vi "Begin.vi"() -> (0 "CameraDevRef 2":T1, 1 "CameraDevRef":T1)   [LabVIEW 2011]
doc: "Called before other user functions, this VI is expected to open initial I/O refnums, load in file data, and do all program initialization. Notice that the <B>error out</B> terminal is simply used for data flow. Wiring it to other structures or subVIs ensures that this VI runs first."
uses:
  <vilib>/Rock Robotics/WPI/Camera/WPI_CameraDevRef.ctl
  <vilib>/Rock Robotics/SystemInterfaces/DIO/FPGA_DIOPWMChannel.ctl
  <vilib>/Rock Robotics/WPI/Joystick/WPI_JoystickDeviceEnum.ctl
  <vilib>/Rock Robotics/SystemInterfaces/AI/FPGA_AIChannel.ctl
  <vilib>/Rock Robotics/SystemInterfaces/DIO/FPGA_DIORelayChannel.ctl
  <vilib>/Rock Robotics/SystemInterfaces/DIO/FPGA_DIOChannel.ctl
  <vilib>/Rock Robotics/SystemInterfaces/AI/FPGA_AIGyroChannel.ctl
  <vilib>/Rock Robotics/WPI/Relay/WPI_RelayDirection.ctl
  <vilib>/Rock Robotics/WPI/Encoder/WPI_EncoderType.ctl
  <vilib>/Rock Robotics/WPI/MotorControl/WPI_MotorControlOpen Victor.vi
  <vilib>/Rock Robotics/WPI/MotorControl/WPI_MotorControlOpen Jaguar.vi
  Robot Global Data.vi
  <vilib>/Utility/file.llb/Read From Spreadsheet File (DBL).vi
  <vilib>/Rock Robotics/WPI/Counter/WPI_CounterDigitalInputToDigitalSource.vi
  <vilib>/Rock Robotics/SystemInterfaces/Typedef/FPGA_TypedefDigitalModule.ctl
  <vilib>/Rock Robotics/SystemInterfaces/Typedef/FPGA_TypedefAnalogModule.ctl
panel:
  out "Path and file":string
  in  "Balls In Robot At Start":dbl=2.0
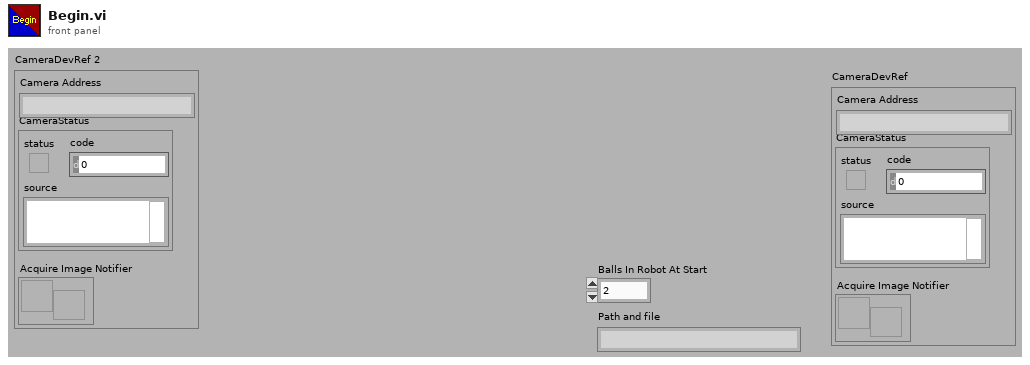
[diagram p1: front panel]
types:
  T1 = typedef "WPI_CameraDevRef.ctl" = cluster{"Camera Address":string, "CameraStatus":errorcluster, "Acquire Image Notifier":refnum<notifier>}
  T2 = typedef "WPI_EncoderType.ctl" = enum16{"1x", "2x", "4x"}
  T3 = typedef "FPGA_DIOChannel.ctl" = enum8{"DIO 1", "DIO 2", "DIO 3", "DIO 4", "DIO 5", "DIO 6", "DIO 7", "DIO 8", "DIO 9", "DIO 10", "DIO 11", "DIO 12", "DIO 13", "DIO 14", "Invalid"}
  T4 = typedef "FPGA_DIORelayChannel.ctl" = enum8{"Relay 1", "Relay 2", "Relay 3", "Relay 4", "Relay 5", "Relay 6", "Relay 7", "Relay 8", "Invalid"}
  T5 = typedef "WPI_RelayDirection.ctl" = enum16{"Both directions", "Forward only", "Reverse only"}
  T6 = typedef "FPGA_AIGyroChannel.ctl" = enum8{"AI 1", "AI 2", "Invalid"}
  T7 = typedef "FPGA_DIOPWMChannel.ctl" = enum8{"PWM 1", "PWM 2", "PWM 3", "PWM 4", "PWM 5", "PWM 6", "PWM 7", "PWM 8", "PWM 9", "PWM 10", "Invalid"}
  T8 = typedef "FPGA_AIChannel.ctl" = enum8{"AI 1", "AI 2", "AI 3", "AI 4", "AI 5", "AI 6", "AI 7", "AI 8", "Invalid"}
  T9 = typedef "WPI_JoystickDeviceEnum.ctl" = enum16{"USB 1", "USB 2", "USB 3", "USB 4", "Kinect 1", "Kinect 2"}
  T10 = typedef "WPI_CameraImageSize.ctl" = enum16{"640x480", "320x240", "160x120"}
  T11 = cluster{"fps":i32, "compression":i32, "Image Size":T10}
  T12 = typedef "WPI_MotorControlDeviceRef.ctl" = cluster{"DeviceStatus":errorcluster, "Type":enum16{"PWM", "CAN"}, "PWM":cluster{"Digital Module":T13, "PWM Channel":T7, "DeadBand":T14}, "CAN":cluster{"Device Number":u8, "Control Mode":T15, "Semaphore":T16, "Max Vout":dbl}, "Invert":bool, "TransformRef":T17, "InvTransformRef":T17}
  T13 = typedef "FPGA_TypedefDigitalModule.ctl" = enum16{"Digital Module 1", "Digital Module 2"}
  T14 = typedef "WPI_PWMDeadband.ctl" = cluster{"Name":string, "maxPositivePwm":i32, "minPositivePwm":i32, "centerPwm":i32, "maxNegativePwm":i32, "minNegativePwm":i32, "angularRange":u16}
  T15 = typedef "WPI_CANJaguar_ControlMode.ctl" = enum8{"Percent VBus", "Current", "Speed", "Position", "Voltage"}
  T16 = typedef "Semaphore RefNum" = refnum<k1>
  T17 = typedef "WPI_PWMTransform_ConPane.ctl" = refnum<vi>
  T18 = typedef "WPI_ServoDeviceRef.ctl" = cluster{"DeviceStatus":errorcluster, "Digital Module":T13, "PWM Channel":T7, "DeadBand":T14}
  T19 = typedef "WPI_AnalogChannelDevRef.ctl" = cluster{"DevStatus":errorcluster, "Analog Module":T20, "Analog Channel":T8}
  T20 = typedef "FPGA_TypedefAnalogModule.ctl" = enum16{"Analog Module 1", "Analog Module 2"}
  T21 = typedef "WPI_CameraWhite Balance Values.ctl" = enum16{"Auto", "Fixed indoor", "Fixed outdoor 1", "Fixed outdoor 2", "Fixed fluorescent 1", "Fixed fluorescent 2", "Hold current"}
  T22 = typedef "WPI_JoystickDevRef.ctl" = cluster{"Device":T9}
  T23 = typedef "WPI_RelayDevRef.ctl" = cluster{"DevStatus":errorcluster, "Relay Channel":T4, "Digital Module":T13, "Relay Direction":T5}
  T24 = typedef "WPI_CameraExposure Values.ctl" = enum16{"Auto", "Flicker-free 50 Hz", "Flicker-free 60 Hz", "Hold current"}
  T25 = typedef "WPI_DigitalInputDevRef.ctl" = cluster{"DevStatus":errorcluster, "DIO Channel":T3, "Digital Module":T13}
  T26 = typedef "FPGA_CounterEncoderSourceConvertionLVSourceType.ctl" = cluster{"DevStatus":errorcluster, "AnalogTriggerMode?":bool, "DigitalMode":cluster{"Digital Module":T13, "DIO Channel":T27}, "AnalogTriggerMode":cluster{"AnalogTriggerIndex":T28, "OutputType":T29}}
  T27 = typedef "FPGA_DIODigitalSourceChannel.ctl" = enum8{"DIO 1", "DIO 2", "DIO 3", "DIO 4", "DIO 5", "DIO 6", "DIO 7", "DIO 8", "DIO 9", "DIO 10", "DIO 11", "DIO 12", "DIO 13", "DIO 14", "Disabled"}
  T28 = typedef "FPGA_AnalogTriggerIndex.ctl" = enum8{"Trig 0", "Trig 1", "Trig 2", "Trig 3", "Trig 4", "Trig 5", "Trig 6", "Trig 7", "Invalid"}
  T29 = typedef "FPGA_AnalogTriggerOutType.ctl" = enum16{"InWindow", "TriggerState", "Rising", "Falling"}
  T30 = typedef "WPI_EncoderDevRef.ctl" = cluster{"DevStatus":errorcluster, "EncoderIndex":T31, "CounterIndex":T32, "DistancePerCount":dbl, "Decoding Type":T2}
  T31 = typedef "FPGA_EncoderIdx.ctl" = enum8{"Enc 0", "Enc 1", "Enc 2", "Enc 3", "Invalid"}
  T32 = typedef "FPGA_CounterCtrSystemIndex.ctl" = enum8{"Ctr 0", "Ctr 1", "Ctr 2", "Ctr 3", "Ctr 4", "Ctr 5", "Ctr 6", "Ctr 7", "Invalid"}
  T33 = typedef "WPI_GyroDevRef.ctl" = cluster{"DevStatus":errorcluster, "Analog Module":T20, "Analog Channel":T8, "Offset":dbl, "Gain (VoltsPerDegree/Second)":dbl}
  T34 = typedef "WPI_UltrasonicDeviceRef.ctl" = cluster{"DevStatus":errorcluster, "Ping Digital Module":T13, "Echo Digital Module":T13, "Ping Channel":T3, "Echo Channel":T3, "CntIndex":T32}
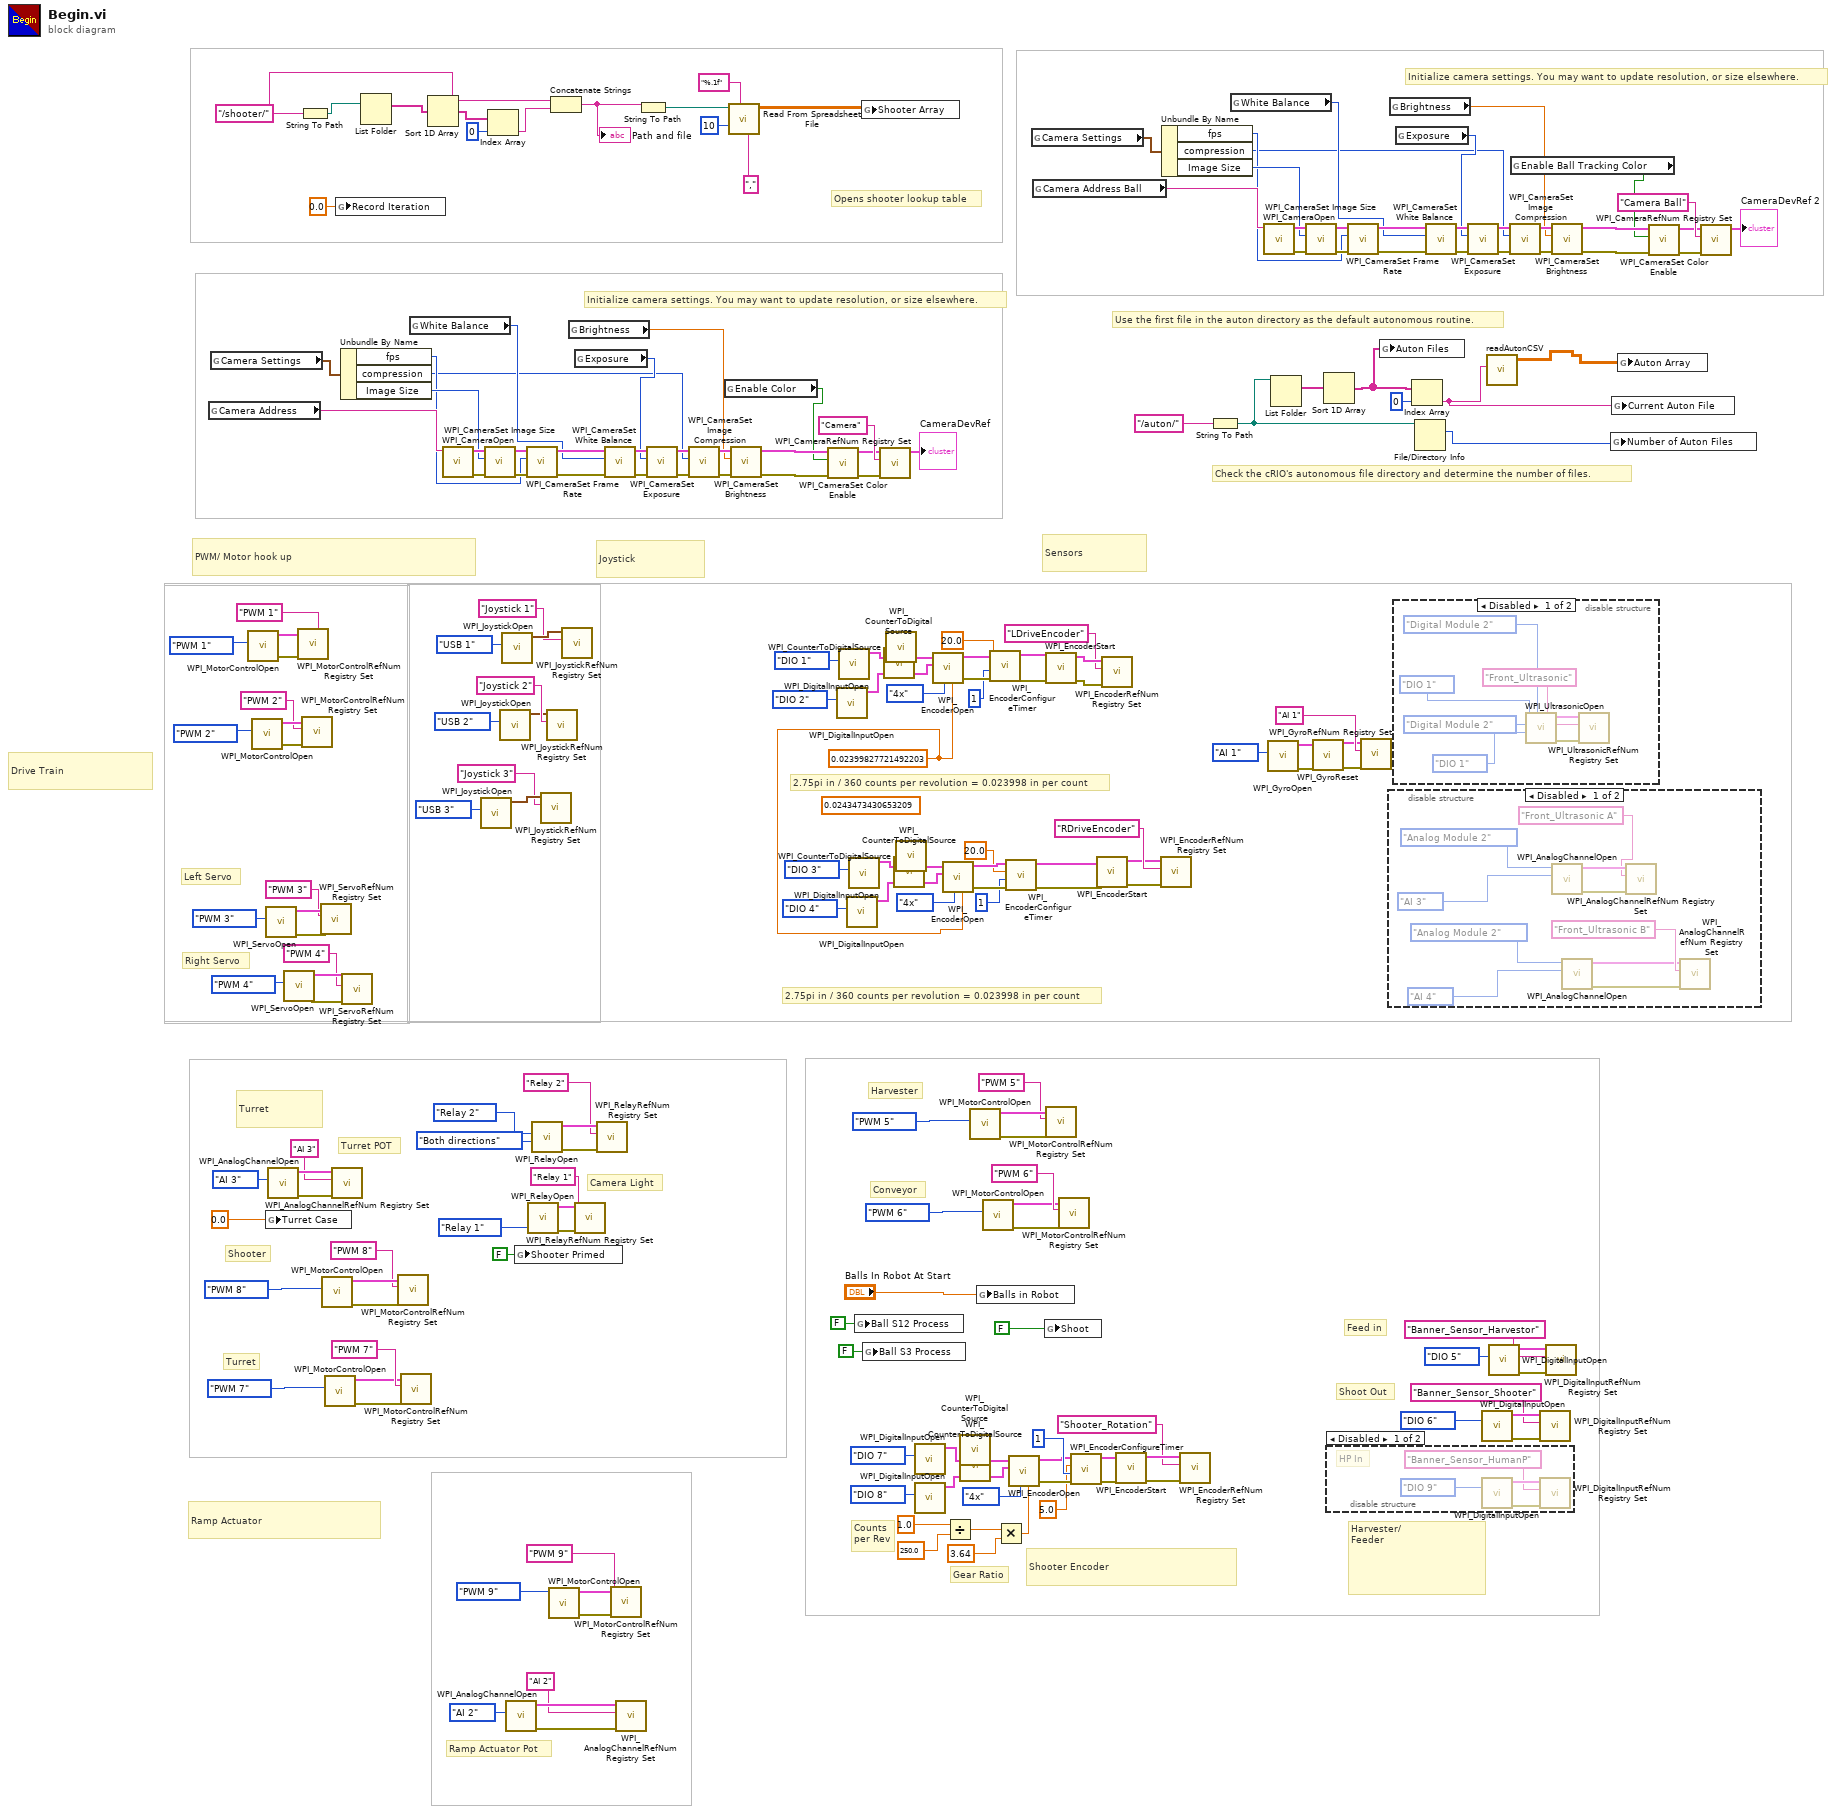
[diagram p0: block diagram]
diagram:
  (unwired) 0.0243473430653209 ("DistancePerCount")
  w49 = 0.02399827721492203 ("DistancePerCount")
  w99 = "/shooter/" ("string")
  # "Shooter Encoder"
  # "Counts\nper Rev"
  # "Gear Ratio"
  # "Initialize camera settings. You may want to update resolution, or size elsewhere."
  # "Check the cRIO's autonomous file directory and determine the number of files."
  # "Use the first file in the auton directory as the default autonomous routine."
  # "2.75pi in / 360 counts per revolution = 0.023998 in per count"
  # "2.75pi in / 360 counts per revolution = 0.023998 in per count"
  # "Opens shooter lookup table"
  # "Shoot Out"
  # "Feed in"
  # "Harvester"
  # "Conveyor"
  # "Shooter"
  # "Initialize camera settings. You may want to update resolution, or size elsewhere."
  # "Camera Light"
  # "Ramp Actuator Pot"
  # "Turret POT"
  # "Turret"
  # "Right Servo"
  # "Left Servo"
  # "Harvester/\nFeeder"
  # "Turret"
  # "Ramp Actuator"
  # "Drive Train"
  # "Sensors"
  # "Joystick"
  # "PWM/ Motor hook up"
  n1 = global read "Robot Global Data.vi" "Camera Address"() -> (w152:string)
  n2 = global read "Robot Global Data.vi" "Camera Settings"() -> (w151:T11)
  n3 = call-poly <vilib>:"WPI_MotorControlOpen.vi"("PWM Channel"=FPGA_DIOPWMChannel."PWM 1") -> ("error out"=w192:errorcluster, "MotorControlDeviceRef"=w194:T12)  [unwired: 9 in]
  n4 = call-poly <vilib>:"WPI_MotorControlOpen.vi"("PWM Channel"=FPGA_DIOPWMChannel."PWM 2") -> ("error out"=w190:errorcluster, "MotorControlDeviceRef"=w188:T12)  [unwired: 9 in]
  n5 = call <vilib>:"WPI_ServoOpen.vi"("PWM Channel"=FPGA_DIOPWMChannel."PWM 3") -> ("error out"=w205:errorcluster, "ServoDeviceRef"=w210:T18)  [unwired: 9 in]
  n6 = global write "Robot Global Data.vi" "Turret Case"(0.0 ("Return To Home Case")) -> ()
  n7 = call <vilib>:"WPI_AnalogChannelOpen.vi"("Analog Channel"=FPGA_AIChannel."AI 3") -> ("error out"=w181:errorcluster, "AIDeviceRef"=w182:T19)  [unwired: 9 in]
  n8 = call <vilib>:"WPI_ServoOpen.vi"("PWM Channel"=FPGA_DIOPWMChannel."PWM 4") -> ("error out"=w204:errorcluster, "ServoDeviceRef"=w208:T18)  [unwired: 9 in]
  n9 = call <vilib>:"WPI_MotorControlRefNum Registry Set.vi"("error in (no error)"=w192, "refnum name"="PWM 1", "MotorControlDevRef"=w194) -> ()  [unwired: 7 in, 2 out]
  n10 = String To Path(string=w99) -> (path=w108:path)
  n11 = call <vilib>:"WPI_MotorControlRefNum Registry Set.vi"("error in (no error)"=w190, "refnum name"="PWM 2", "MotorControlDevRef"=w188) -> ()  [unwired: 7 in, 2 out]
  n12 = call <vilib>:"WPI_ServoRefNum Registry Set.vi"("error in (no error)"=w205, "refnum name"="PWM 3", "ServoDeviceRef"=w210) -> ()  [unwired: 7 in, 2 out]
  n13 = call-poly <vilib>:"WPI_MotorControlOpen.vi"("PWM Channel"=FPGA_DIOPWMChannel."PWM 8") -> ("error out"=w135:errorcluster, "MotorControlDeviceRef"=w137:T12)  [unwired: 9 in]
  n14 = call-poly <vilib>:"WPI_MotorControlOpen.vi"("PWM Channel"=FPGA_DIOPWMChannel."PWM 7") -> ("error out"=w186:errorcluster, "MotorControlDeviceRef"=w184:T12)  [unwired: 9 in]
  n15 = call <vilib>:"WPI_AnalogChannelRefNum Registry Set.vi"("error in (no error)"=w181, "refnum name"="AI 3", "AIDeviceRef"=w182) -> ()  [unwired: 7 in, 2 out]
  n16 = global write "Robot Global Data.vi" "Record Iteration"(0.0 ("Record Iteration")) -> ()
  n17 = Unbundle By Name(w151) -> ("fps"=w149:i32, "compression"=w146:i32, "Image Size"=w150:T10)
  n18 = call <vilib>:"WPI_ServoRefNum Registry Set.vi"("error in (no error)"=w204, "refnum name"="PWM 4", "ServoDeviceRef"=w208) -> ()  [unwired: 7 in, 2 out]
  n19 = List Folder(path=w108) -> (filenames=w107:string[])  [unwired: 1 in, 5 out]
  n20 = call <vilib>:"WPI_MotorControlRefNum Registry Set.vi"("error in (no error)"=w135, "refnum name"="PWM 8", "MotorControlDevRef"=w137) -> ()  [unwired: 7 in, 2 out]
  n21 = call <vilib>:"WPI_MotorControlRefNum Registry Set.vi"("error in (no error)"=w186, "refnum name"="PWM 7", "MotorControlDevRef"=w184) -> ()  [unwired: 7 in, 2 out]
  n22 = global read "Robot Global Data.vi" "White Balance"() -> (w148:T21)
  n23 = Sort 1D Array(array=w107) -> (sorted array=w106:string[])
  n24 = call <vilib>:"WPI_CameraOpen.vi"("Camera Address"=w152) -> ("error out"=w158:errorcluster, "CameraDevRef"=w159:T1)  [unwired: 1 in, 8 out]
  n25 = call <vilib>:"WPI_JoystickOpen.vi"("JoystickDevice"=WPI_JoystickDeviceEnum."USB 3") -> ("JoystickDevRef"=w197:T22)  [unwired: 10 in]
  n26 = call <vilib>:"WPI_CameraSet Image Size.vi"("error in (no error)"=w158, "Image Size"=w150, "CameraDevRef"=w159) -> ("error out"=w157:errorcluster, "CameraDevRef Out"=w160:T1)  [unwired: 7 out]
  n27 = Index Array(array=w106, index=0) -> (element=w98:string)
  n28 = call <vilib>:"WPI_JoystickOpen.vi"("JoystickDevice"=WPI_JoystickDeviceEnum."USB 2") -> ("JoystickDevRef"=w200:T22)  [unwired: 10 in]
  n29 = call <vilib>:"WPI_JoystickOpen.vi"("JoystickDevice"=WPI_JoystickDeviceEnum."USB 1") -> ("JoystickDevRef"=w203:T22)  [unwired: 10 in]
  n30 = call <vilib>:"WPI_AnalogChannelOpen.vi"("Analog Channel"=FPGA_AIChannel."AI 2") -> ("error out"=w176:errorcluster, "AIDeviceRef"=w177:T19)  [unwired: 9 in]
  n31 = global write "Robot Global Data.vi" "Shooter Primed"(FALSE ("Ball S3 Process")) -> ()
  n32 = call <vilib>:"WPI_CameraSet Frame Rate.vi"("error in (no error)"=w157, "Frame Rate (fps)"=w149, "CameraDevRef"=w160) -> ("error out"=w156:errorcluster, "CameraDevRef Out"=w162:T1)  [unwired: 7 out]
  n33 = call <vilib>:"WPI_RelayOpen.vi"("Relay Channel"=FPGA_DIORelayChannel."Relay 1") -> ("error out"=w169:errorcluster, "RelayDevRef"=w168:T23)  [unwired: 9 in]
  n34 = call <vilib>:"WPI_RelayOpen.vi"("Relay Direction"=WPI_RelayDirection."Both directions", "Relay Channel"=FPGA_DIORelayChannel."Relay 2") -> ("error out"=w93:errorcluster, "RelayDevRef"=w94:T23)  [unwired: 8 in]
  n35 = call <vilib>:"WPI_JoystickRefNum Registry Set.vi"("refnum name"="Joystick 3", "JoystickDevRef"=w197) -> ()  [unwired: 8 in, 2 out]
  n36 = call <vilib>:"WPI_JoystickRefNum Registry Set.vi"("refnum name"="Joystick 2", "JoystickDevRef"=w200) -> ()  [unwired: 8 in, 2 out]
  n37 = call-poly <vilib>:"WPI_MotorControlOpen.vi"("PWM Channel"=FPGA_DIOPWMChannel."PWM 9") -> ("error out"=w172:errorcluster, "MotorControlDeviceRef"=w173:T12)  [unwired: 9 in]
  n38 = Concatenate Strings(w99, w98) -> (w101:string)
  "Path and file" <- w101
  n39 = call <vilib>:"WPI_JoystickRefNum Registry Set.vi"("refnum name"="Joystick 1", "JoystickDevRef"=w203) -> ()  [unwired: 8 in, 2 out]
  n40 = global read "Robot Global Data.vi" "Brightness"() -> (w145:dbl)
  n41 = global read "Robot Global Data.vi" "Exposure"() -> (w147:T24)
  n42 = call <vilib>:"WPI_RelayRefNum Registry Set.vi"("error in (no error)"=w169, "refnum name"="Relay 1", "RelayDevRef"=w168) -> ()  [unwired: 7 in, 2 out]
  n43 = call <vilib>:"WPI_RelayRefNum Registry Set.vi"("error in (no error)"=w93, "refnum name"="Relay 2", "RelayDevRef"=w94) -> ()  [unwired: 7 in, 2 out]
  n44 = call <vilib>:"WPI_CameraSet White Balance.vi"("error in (no error)"=w156, "White Balance"=w148, "CameraDevRef"=w162) -> ("error out"=w155:errorcluster, "CameraDevRef Out"=w161:T1)  [unwired: 7 out]
  n45 = call <vilib>:"WPI_MotorControlRefNum Registry Set.vi"("error in (no error)"=w172, "refnum name"="PWM 9", "MotorControlDevRef"=w173) -> ()  [unwired: 7 in, 2 out]
  n46 = call <vilib>:"WPI_AnalogChannelRefNum Registry Set.vi"("error in (no error)"=w176, "refnum name"="AI 2", "AIDeviceRef"=w177) -> ()  [unwired: 7 in, 2 out]
  n47 = String To Path(string=w101) -> (path=w100:path)
  n48 = call <vilib>:"WPI_CameraSet Exposure.vi"("error in (no error)"=w155, "Exposure"=w147, "CameraDevRef"=w161) -> ("error out"=w154:errorcluster, "CameraDevRef Out"=w164:T1)  [unwired: 7 out]
  n49 = call <vilib>:"WPI_CameraSet Image Compression.vi"("error in (no error)"=w154, "Compression"=w146, "CameraDevRef"=w164) -> ("error out"=w153:errorcluster, "CameraDevRef Out"=w163:T1)  [unwired: 7 out]
  n50 = global read "Robot Global Data.vi" "Enable Color"() -> (w140:bool)
  n51 = call-poly <vilib>:"Read From Spreadsheet File.vi"("delimiter (\\t)"="," ("delimiter (\\t)"), "format (%.3f)"="%.1f", "number of rows (all:-1)"=10, "file path (dialog if empty)"=w100) -> ("all rows"=w97:dbl[][])  [unwired: 1 in, 6 out]
  n52 = call <vilib>:"WPI_CameraSet Brightness.vi"("error in (no error)"=w153, "Brightness"=w145, "CameraDevRef"=w163) -> ("error out"=w143:errorcluster, "CameraDevRef Out"=w144:T1)  [unwired: 7 out]
  n53 = call <vilib>:"WPI_CameraSet Color Enable.vi"("error in (no error)"=w143, "Color Enabled"=w140, "CameraDevRef"=w144) -> ("error out"=w141:errorcluster, "CameraDevRef Out"=w142:T1)  [unwired: 7 in]
  n54 = call <vilib>:"WPI_DigitalInputOpen.vi"("DIO Channel"=FPGA_DIOChannel."DIO 2") -> ("DigitalInputDevRef"=w85:T25)  [unwired: 9 in, 1 out]
  n55 = call <vilib>:"WPI_DigitalInputOpen.vi"("DIO Channel"=FPGA_DIOChannel."DIO 1") -> ("DigitalInputDevRef"=w82:T25)  [unwired: 9 in, 1 out]
  n56 = call <vilib>:"WPI_DigitalInputOpen.vi"("DIO Channel"=FPGA_DIOChannel."DIO 4") -> ("DigitalInputDevRef"=w76:T25)  [unwired: 9 in, 1 out]
  n57 = call <vilib>:"WPI_DigitalInputOpen.vi"("DIO Channel"=FPGA_DIOChannel."DIO 3") -> ("DigitalInputDevRef"=w79:T25)  [unwired: 9 in, 1 out]
  n58 = global write "Robot Global Data.vi" "Ball S12 Process"(FALSE ("Ball S12 Process")) -> ()
  n59 = global write "Robot Global Data.vi" "Shooter Array"(w97) -> ()
  n60 = global write "Robot Global Data.vi" "Ball S3 Process"(FALSE ("Ball S3 Process")) -> ()
  n61 = call <vilib>:"WPI_CameraRefNum Registry Set.vi"("error in (no error)"=w141, "refnum name"="Camera", "CameraDevRef"=w142) -> ("CameraDevRef"=→"CameraDevRef":T1)  [unwired: 8 out]
  n62 = call-poly <vilib>:"WPI_CounterToDigitalSource.vi"("DigitalInputDevRef"=w85) -> ("Digital Source"=w86:T26)  [unwired: 6 in]
  n63 = call-poly <vilib>:"WPI_CounterToDigitalSource.vi"("DigitalInputDevRef"=w82) -> ("Digital Source"=w81:T26)  [unwired: 6 in]
  n64 = call-poly <vilib>:"WPI_CounterToDigitalSource.vi"("DigitalInputDevRef"=w76) -> ("Digital Source"=w75:T26)  [unwired: 6 in]
  n65 = call-poly <vilib>:"WPI_CounterToDigitalSource.vi"("DigitalInputDevRef"=w79) -> ("Digital Source"=w80:T26)  [unwired: 6 in]
  n66 = call <vilib>:"WPI_DigitalInputOpen.vi"("DIO Channel"=FPGA_DIOChannel."DIO 7") -> ("DigitalInputDevRef"=w33:T25)  [unwired: 9 in, 1 out]
  n67 = call <vilib>:"WPI_DigitalInputOpen.vi"("DIO Channel"=FPGA_DIOChannel."DIO 8") -> ("DigitalInputDevRef"=w36:T25)  [unwired: 9 in, 1 out]
  n68 = call <vilib>:"WPI_EncoderOpen.vi"("DistancePerCount"=w49, "Decoding Type"=WPI_EncoderType."4x", "BSource"=w86, "ASource"=w81) -> ("error out"=w53:errorcluster, "EncoderDevRef"=w56:T30)  [unwired: 6 in]
  n69 = call <vilib>:"WPI_EncoderOpen.vi"("DistancePerCount"=w49, "Decoding Type"=WPI_EncoderType."4x", "BSource"=w75, "ASource"=w80) -> ("error out"=w72:errorcluster, "EncoderDevRef"=w71:T30)  [unwired: 6 in]
  n70 = Divide(x=1.0, y=250.0) -> (x/y=w30:dbl)
  n71 = call-poly <vilib>:"WPI_CounterToDigitalSource.vi"("DigitalInputDevRef"=w33) -> ("Digital Source"=w32:T26)  [unwired: 6 in]
  n72 = call-poly <vilib>:"WPI_CounterToDigitalSource.vi"("DigitalInputDevRef"=w36) -> ("Digital Source"=w37:T26)  [unwired: 6 in]
  n73 = call-poly <vilib>:"WPI_MotorControlOpen.vi"("PWM Channel"=FPGA_DIOPWMChannel."PWM 5") -> ("error out"=w131:errorcluster, "MotorControlDeviceRef"=w133:T12)  [unwired: 9 in]
  n74 = global write "Robot Global Data.vi" "Balls in Robot"("Balls In Robot At Start") -> ()
  n75 = call-poly <vilib>:"WPI_MotorControlOpen.vi"("PWM Channel"=FPGA_DIOPWMChannel."PWM 6") -> ("error out"=w130:errorcluster, "MotorControlDeviceRef"=w128:T12)  [unwired: 9 in]
  n76 = call <vilib>:"WPI_EncoderConfigureTimer.vi"("error in (no error)"=w53, "Number Samples to Average"=u8 1, "Minimum Rate"=20.0, "EncoderDevRef"=w56) -> ("error out"=w54:errorcluster, "EncoderDevRef"=w55:T30)  [unwired: 6 in]
  n77 = Multiply(x=w30, y=3.64) -> (x*y=w28:dbl)
  n78 = call <vilib>:"WPI_EncoderConfigureTimer.vi"("error in (no error)"=w72, "Number Samples to Average"=u8 1, "Minimum Rate"=20.0, "EncoderDevRef"=w71) -> ("error out"=w68:errorcluster, "EncoderDevRef"=w69:T30)  [unwired: 6 in]
  n79 = call <vilib>:"WPI_EncoderOpen.vi"("DistancePerCount"=w28, "Decoding Type"=WPI_EncoderType."4x", "BSource"=w37, "ASource"=w32) -> ("error out"=w40:errorcluster, "EncoderDevRef"=w41:T30)  [unwired: 6 in]
  n80 = global read "Robot Global Data.vi" "Camera Settings"() -> (w13:T11)
  n81 = global read "Robot Global Data.vi" "Camera Address Ball"() -> (w14:string)
  n82 = global write "Robot Global Data.vi" "Shoot"(FALSE ("Ball S12 Process")) -> ()
  n83 = call <vilib>:"WPI_EncoderStart.vi"("error in (no error)"=w54, "EncoderDevRef"=w55) -> ("error out"=w89:errorcluster, "EncoderDevRef"=w88:T30)  [unwired: 8 in]
  n84 = call <vilib>:"WPI_MotorControlRefNum Registry Set.vi"("error in (no error)"=w131, "refnum name"="PWM 5", "MotorControlDevRef"=w133) -> ()  [unwired: 7 in, 2 out]
  n85 = call <vilib>:"WPI_MotorControlRefNum Registry Set.vi"("error in (no error)"=w130, "refnum name"="PWM 6", "MotorControlDevRef"=w128) -> ()  [unwired: 7 in, 2 out]
  n86 = call <vilib>:"WPI_EncoderConfigureTimer.vi"("error in (no error)"=w40, "Number Samples to Average"=u8 1, "Minimum Rate"=5.0, "EncoderDevRef"=w41) -> ("error out"=w44:errorcluster, "EncoderDevRef"=w43:T30)  [unwired: 6 in]
  n87 = call <vilib>:"WPI_EncoderStart.vi"("error in (no error)"=w68, "EncoderDevRef"=w69) -> ("error out"=w66:errorcluster, "EncoderDevRef"=w67:T30)  [unwired: 8 in]
  n88 = call <vilib>:"WPI_EncoderRefNum Registry Set.vi"("error in (no error)"=w89, "refnum name"="LDriveEncoder", "EncoderDevRef"=w88) -> ()  [unwired: 7 in, 2 out]
  n89 = call <vilib>:"WPI_EncoderStart.vi"("error in (no error)"=w44, "EncoderDevRef"=w43) -> ("error out"=w46:errorcluster, "EncoderDevRef"=w45:T30)  [unwired: 8 in]
  n90 = call <vilib>:"WPI_EncoderRefNum Registry Set.vi"("error in (no error)"=w66, "refnum name"="RDriveEncoder", "EncoderDevRef"=w67) -> ()  [unwired: 7 in, 2 out]
  n91 = Unbundle By Name(w13) -> ("fps"=w11:i32, "compression"=w8:i32, "Image Size"=w12:T10)
  n92 = call <vilib>:"WPI_EncoderRefNum Registry Set.vi"("error in (no error)"=w46, "refnum name"="Shooter_Rotation", "EncoderDevRef"=w45) -> ()  [unwired: 7 in, 2 out]
  n93 = String To Path(string="/auton/") -> (path=w61:path)
  n94 = global read "Robot Global Data.vi" "White Balance"() -> (w10:T21)
  n95 = call <vilib>:"WPI_CameraOpen.vi"("Camera Address"=w14) -> ("error out"=w20:errorcluster, "CameraDevRef"=w21:T1)  [unwired: 1 in, 8 out]
  n96 = call <vilib>:"WPI_GyroOpen.vi"("Analog Channel"=FPGA_AIGyroChannel."AI 1") -> ("error out"=w111:errorcluster, "GyroDevRef"=w112:T33)  [unwired: 8 in, 1 out]
  n97 = List Folder(path=w61) -> (filenames=w60:string[])  [unwired: 1 in, 5 out]
  n98 = call <vilib>:"WPI_CameraSet Image Size.vi"("error in (no error)"=w20, "Image Size"=w12, "CameraDevRef"=w21) -> ("error out"=w19:errorcluster, "CameraDevRef Out"=w22:T1)  [unwired: 7 out]
  n99 = call <vilib>:"WPI_GyroReset.vi"("error in (no error)"=w111, "GyroDevRef"=w112) -> ("error out"=w110:errorcluster, "GyroDevRef"=w109:T33)  [unwired: 8 in]
  n100 = Sort 1D Array(array=w60) -> (sorted array=w58:string[])
  n101 = disable-structure shown="Disabled" {
    frame Disabled {
      # "HP In"
      n102 = call <vilib>:"WPI_DigitalInputOpen.vi"("DIO Channel"=FPGA_DIOChannel."DIO 9") -> ("error out"=w214:errorcluster, "DigitalInputDevRef"=w213:T25)  [unwired: 9 in]
      n103 = call <vilib>:"WPI_DigitalInputRefNum Registry Set.vi"("error in (no error)"=w214, "refnum name"="Banner_Sensor_HumanP", "DigitalInputDevRef"=w213) -> ()  [unwired: 7 in, 2 out]
    }
    frame Enabled {
    }
  }
  n104 = call <vilib>:"WPI_CameraSet Frame Rate.vi"("error in (no error)"=w19, "Frame Rate (fps)"=w11, "CameraDevRef"=w22) -> ("error out"=w18:errorcluster, "CameraDevRef Out"=w24:T1)  [unwired: 7 out]
  n105 = call <vilib>:"WPI_GyroRefNum Registry Set.vi"("error in (no error)"=w110, "refnum name"="AI 1", "GyroDevRef"=w109) -> ()  [unwired: 7 in, 2 out]
  n106 = global write "Robot Global Data.vi" "Auton Files"(w58) -> ()
  n107 = disable-structure shown="Disabled" {
    frame Disabled {
      n108 = call <vilib>:"WPI_AnalogChannelOpen.vi"("Analog Channel"=FPGA_AIChannel."AI 3", "Analog Module (Module 1)"=FPGA_TypedefAnalogModule."Analog Module 2") -> ("error out"=w221:errorcluster, "AIDeviceRef"=w220:T19)  [unwired: 8 in]
      n109 = call <vilib>:"WPI_AnalogChannelOpen.vi"("Analog Channel"=FPGA_AIChannel."AI 4", "Analog Module (Module 1)"=FPGA_TypedefAnalogModule."Analog Module 2") -> ("error out"=w216:errorcluster, "AIDeviceRef"=w217:T19)  [unwired: 8 in]
      n110 = call <vilib>:"WPI_AnalogChannelRefNum Registry Set.vi"("error in (no error)"=w221, "refnum name"="Front_Ultrasonic A", "AIDeviceRef"=w220) -> ()  [unwired: 7 in, 2 out]
      n111 = call <vilib>:"WPI_AnalogChannelRefNum Registry Set.vi"("error in (no error)"=w216, "refnum name"="Front_Ultrasonic B", "AIDeviceRef"=w217) -> ()  [unwired: 7 in, 2 out]
    }
    frame Enabled {
    }
  }
  n112 = global read "Robot Global Data.vi" "Brightness"() -> (w7:dbl)
  n113 = disable-structure shown="Disabled" {
    frame Disabled {
      n114 = call <vilib>:"WPI_UltrasonicOpen.vi"("Ping Digital Module (Module 1)"=FPGA_TypedefDigitalModule."Digital Module 2", "Echo DIO Channel"=FPGA_DIOChannel."DIO 1", "Echo Digital Module (Module 1)"=FPGA_TypedefDigitalModule."Digital Module 2", "Ping DIO Channel"=FPGA_DIOChannel."DIO 1") -> ("error out"=w232:errorcluster, "UltrasonicDevRef"=w231:T34)  [unwired: 6 in]
      n115 = call <vilib>:"WPI_UltrasonicRefNum Registry Set.vi"("error in (no error)"=w232, "refnum name"="Front_Ultrasonic", "UltrasonicDevRef"=w231) -> ()  [unwired: 7 in, 2 out]
    }
    frame Enabled {
    }
  }
  n116 = global read "Robot Global Data.vi" "Exposure"() -> (w9:T24)
  n117 = Index Array(array=w58, index=0) -> (element=w63:string)
  n118 = File/Directory Info(path=w61) -> (size=w64:i64)  [unwired: 1 in, 6 out]
  n119 = call <vilib>:"WPI_CameraSet White Balance.vi"("error in (no error)"=w18, "White Balance"=w10, "CameraDevRef"=w24) -> ("error out"=w17:errorcluster, "CameraDevRef Out"=w23:T1)  [unwired: 7 out]
  n120 = call <vilib>:"WPI_CameraSet Exposure.vi"("error in (no error)"=w17, "Exposure"=w9, "CameraDevRef"=w23) -> ("error out"=w16:errorcluster, "CameraDevRef Out"=w26:T1)  [unwired: 7 out]
  n121 = call <vilib>:"WPI_DigitalInputOpen.vi"("DIO Channel"=FPGA_DIOChannel."DIO 6") -> ("error out"=w121:errorcluster, "DigitalInputDevRef"=w120:T25)  [unwired: 9 in]
  n122 = call "readAutonCSV.vi"("AutonFile"=w63) -> ("AutonArray"=w57:dbl[][])  [unwired: 7 in]
  n123 = call <vilib>:"WPI_DigitalInputOpen.vi"("DIO Channel"=FPGA_DIOChannel."DIO 5") -> ("error out"=w124:errorcluster, "DigitalInputDevRef"=w123:T25)  [unwired: 9 in]
  n124 = call <vilib>:"WPI_CameraSet Image Compression.vi"("error in (no error)"=w16, "Compression"=w8, "CameraDevRef"=w26) -> ("error out"=w15:errorcluster, "CameraDevRef Out"=w25:T1)  [unwired: 7 out]
  n125 = global read "Robot Global Data.vi" "Enable Ball Tracking Color"() -> (w2:bool)
  n126 = call <vilib>:"WPI_DigitalInputRefNum Registry Set.vi"("error in (no error)"=w121, "refnum name"="Banner_Sensor_Shooter", "DigitalInputDevRef"=w120) -> ()  [unwired: 7 in, 2 out]
  n127 = call <vilib>:"WPI_DigitalInputRefNum Registry Set.vi"("error in (no error)"=w124, "refnum name"="Banner_Sensor_Harvestor", "DigitalInputDevRef"=w123) -> ()  [unwired: 7 in, 2 out]
  n128 = call <vilib>:"WPI_CameraSet Brightness.vi"("error in (no error)"=w15, "Brightness"=w7, "CameraDevRef"=w25) -> ("error out"=w5:errorcluster, "CameraDevRef Out"=w6:T1)  [unwired: 7 out]
  n129 = global write "Robot Global Data.vi" "Number of Auton Files"(w64) -> ()
  n130 = global write "Robot Global Data.vi" "Current Auton File"(w63) -> ()
  n131 = global write "Robot Global Data.vi" "Auton Array"(w57) -> ()
  n132 = call <vilib>:"WPI_CameraSet Color Enable.vi"("error in (no error)"=w5, "Color Enabled"=w2, "CameraDevRef"=w6) -> ("error out"=w3:errorcluster, "CameraDevRef Out"=w4:T1)  [unwired: 7 in]
  n133 = call <vilib>:"WPI_CameraRefNum Registry Set.vi"("error in (no error)"=w3, "refnum name"="Camera Ball", "CameraDevRef"=w4) -> ("CameraDevRef"=→"CameraDevRef 2":T1)  [unwired: 8 out]
